vi "DatGetTraceNrs.vi"(8 "error in (no error)":errorcluster, 11 "tracename":string) -> (0 "error out":errorcluster, 1 "Par values":dbl[][](array[numeric]), 2 "Par names":string[](array[string])=["Selected ", "Z0 (um)"], 3 "All Traces":string[](array[string]), 4 "Selected Traces":string[](array[string]))   [LabVIEW 2018]
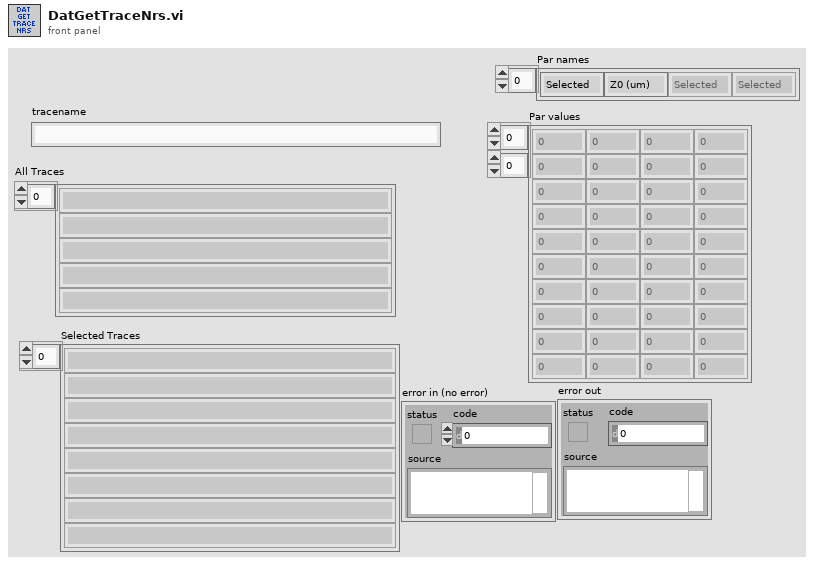
[diagram p1: front panel]
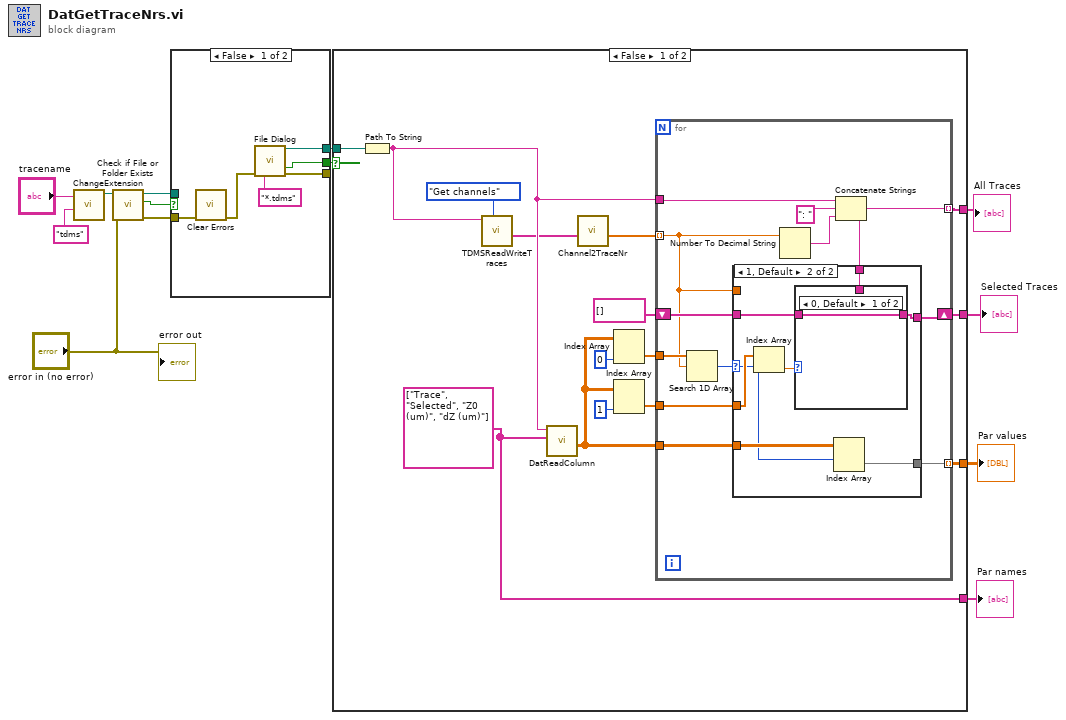
[diagram p0: block diagram]
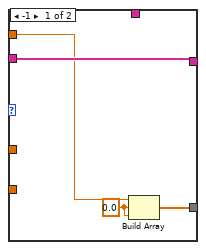
[diagram p2: hidden frame]
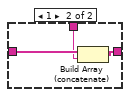
[diagram p3: hidden frame]
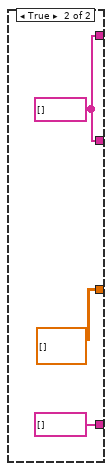
[diagram p4: hidden frame]
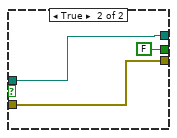
[diagram p5: hidden frame]
diagram:
  n1 = call "ChangeExtension.vi"("extension"="tdms", "file in"="tracename") -> ("Path out"=w6:path)  [unwired: 3 in, 4 out]
  n2 = call <vilib>:"Check if File or Folder Exists.vi"("error in (no error)"="error in (no error)", "path"=w6) -> ("error out"=w8:errorcluster, "file or folder exists?"=w10:bool, "dup path"=w9:path)  [unwired: 7 in]
  n3 = case shown="False" w10 {
    tunnel: [w18 w22] -> w7
    tunnel: [w17 w21] -> _
    tunnel: w9 -> [_ w22]
    tunnel: w8 -> [w16 w21]
    tunnel: [w14 FALSE ("cancelled")] -> w2
    frame False {
      n4 = call <vilib>:"Clear Errors.vi"("error in (no error)"=w16) -> ("error out"=w15:errorcluster)  [unwired: 5 in, 1 out]
      n5 = call "File Dialog"("error in"=w15, "pattern (all files)"="*.tdms") -> ("selected path"=w18:path, "cancelled"=w14:bool, "error out"=w17:errorcluster)  [unwired: 10 in, 1 out]
    }
    frame True {
    }
  }
  n6 = case shown="False" w2 {
    tunnel: [w29 w68] -> w11
    tunnel: w7 -> [w25 _]
    tunnel: [w37 w68] -> w5
    tunnel: [w28 dbl[][] []] -> w4
    tunnel: [w32 string[] []] -> w3
    frame False {
      w32 = string[] ["Trace", "Selected", "Z0 (um)", "dZ (um)"] ("Names")
      n7 = Path To String(path=w25) -> (string=w24:string)
      n8 = call "TDMSReadWriteTraces.vi"("Task"=enum16{"Read", "Write", "Get channels"}."Get channels", "tracename"=w24) -> ("Channels out"=w23:string[])  [unwired: 4 in, 5 out]
      n9 = call "DatReadColumn.vi"("Names"=w32, "tracename"=w24) -> ("Values out"=w27:dbl[][])  [unwired: 5 in, 2 out]
      n10 = call "Channel2TraceNr.vi"("channel names"=w23) -> ("Unique trace numbers"=w35:dbl[])  [unwired: 10 in]
      n11 = Index Array(array=w27, index (col)=0 ("disabled index (col)")) -> (element=w33:dbl[])  [unwired: 1 in]
      n12 = Index Array(array=w27, index (col)=1 ("disabled index (col)")) -> (element=w30:dbl[])  [unwired: 1 in]
      n13 = for {
        tunnel: w24 -> [w47]
        shift-right: [w45] -> w37
        shift-left: string[] [] -> [w46]
        tunnel: w35 -> [w43] mode=indexing
        tunnel: w33 -> [w44]
        tunnel: w30 -> [w39]
        tunnel: [w41] -> w29 mode=indexing
        tunnel: [w40] -> w28 mode=indexing
        tunnel: w27 -> [w38]
        n14 = Search 1D Array(1D array=w44, element=w43) -> (index of element=w42:i32)  [unwired: 1 in]
        n15 = Number To Decimal String(number=w43) -> (decimal integer string=w48:string)  [unwired: 1 in]
        n16 = Concatenate Strings(w47, ": " ("regular expression"), w48) -> (w41:string)
        n17 = case shown="1, Default" w42 {
          selector: w42 -> [_ w54]
          tunnel: w46 -> [w53 w61]
          tunnel: w41 -> [_ w60]
          tunnel: [w53 w59] -> w45
          tunnel: w43 -> [w52 _]
          tunnel: [w51 w55] -> w40
          tunnel: w39 -> [_ w58]
          tunnel: w38 -> [_ w56]
          frame -1 {
            w50 = 0.0 ("element")
            n18 = Build Array(w52, w50, w50) -> (w51:dbl[])
          }
          frame 1, Default {
            n19 = Index Array(array=w58, index=w54) -> (element=w57:dbl)
            n20 = case shown="0, Default" w57 {
              tunnel: w61 -> [w62 w65]
              tunnel: w60 -> [_ w64]
              tunnel: [w62 w63] -> w59
              frame 0, Default {
              }
              frame 1 {
                n21 = Build Array (concatenate)(w65, w64) -> (w63:string[])
              }
            }
            n22 = Index Array(array=w56, index (row)=w54) -> (element=w55:dbl[])  [unwired: 1 in]
          }
        }
      }
    }
    frame True {
      w68 = string[] []
    }
  }
  "Par values" <- w4
  "All Traces" <- w11
  "Selected Traces" <- w5
  "Par names" <- w3
  "error out" <- "error in (no error)"
